vi "cfg upgrade to v2.vi"(11 "Engine Configuration":T11) -> (3 "Engine Configuration out":T1)   [LabVIEW 2013, in "Standard Engine Configuration.lvclass"]
uses:
  Standard Engine Configuration.lvclass
  Supported Timing Sources.ctl
  <vilib>/NI/Tag Bus Module Framework/runtime/error classification.ctl
  Error Actions.ctl
  Engine Configuration.ctl
  Loop Info.ctl
  timing policy.ctl
  Module Specific Configuration.ctl
  Module Decimation.ctl
  Runtime/error responses.ctl
  error options.ctl
  <vilib>/NI/Tag Bus Module Framework/runtime/TBM module execution interface.lvclass
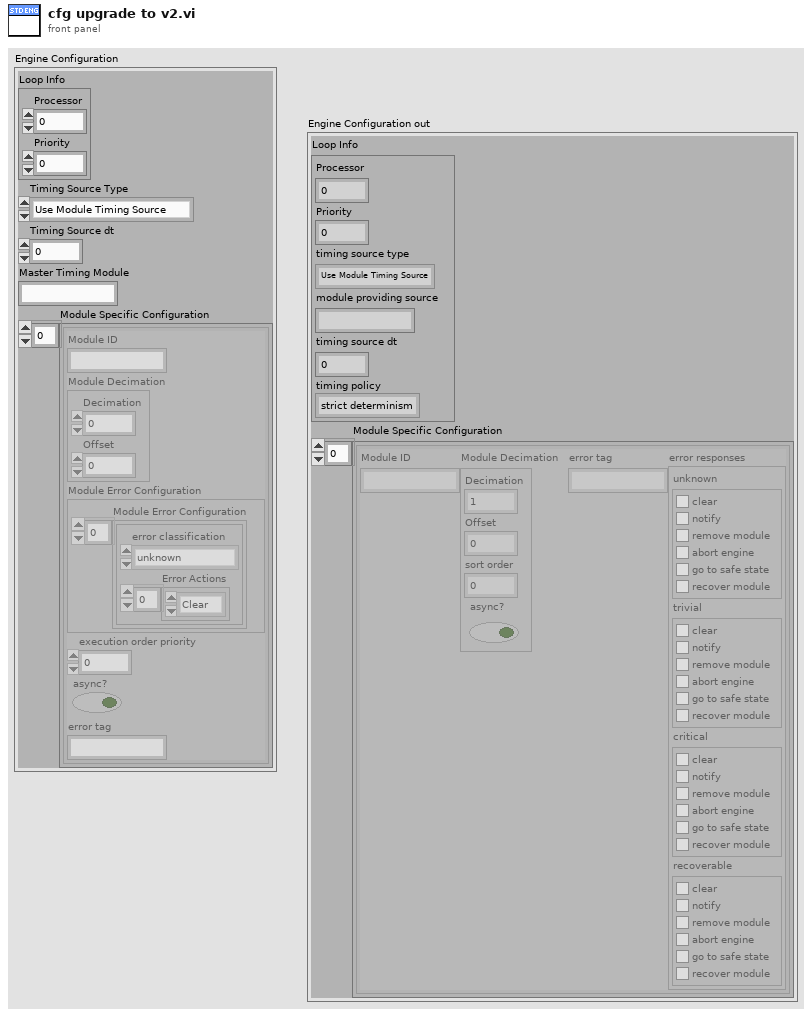
[diagram p1: front panel]
types:
  T1 = typedef "Standard Engine Configuration.lvclass/Engine Configuration.ctl" = cluster{"Loop Info":T2, "Module Specific Configuration":T5[]}
  T2 = typedef "Standard Engine Configuration.lvclass/Loop Info.ctl" = cluster{"Processor":i32, "Priority":i32, "timing source type":T3, "module providing source":string, "timing source dt":u32, "timing policy":T4}
  T3 = typedef "Standard Engine Configuration.lvclass/Supported Timing Sources.ctl" = enum16{"Use Module Timing Source", "1 kHz Clock", "1 MHz Clock", "Synchronize to Scan Engine"}
  T4 = typedef "Standard Engine Configuration.lvclass/timing policy.ctl" = enum16{"strict determinism", "nonblocking", "nondeterministic inline"}
  T5 = typedef "Standard Engine Configuration.lvclass/Module Specific Configuration.ctl" = cluster{"Module ID":string, "Module Decimation":T6, "error tag":string, "error responses":T7}
  T6 = typedef "Standard Engine Configuration.lvclass/Module Decimation.ctl" = cluster{"Decimation":u16, "Offset":u16, "sort order":i32, "async?":bool}
  T7 = typedef "Standard Engine Configuration.lvclass/error responses.ctl" = cluster{"unknown":T8, "trivial":T8, "critical":T8, "recoverable":T8}
  T8 = typedef "Standard Engine Configuration.lvclass/error options.ctl" = cluster{"clear":bool, "notify":bool, "remove module":bool, "abort engine":bool, "go to safe state":bool, "recover module":bool}
  T9 = typedef "TBM module execution interface.lvclass/error classification.ctl" = enum16{"unknown", "none", "trivial", "recoverable", "critical"}
  T10 = typedef "Standard Engine Configuration.lvclass/Error Actions.ctl" = enum16{"Clear", "Notify", "Stop Component", "Stop Engine", "Safe State", "Attempt Recovery"}
  T11 = cluster{"Loop Info":cluster{"Processor":i32, "Priority":i32}, "Timing Source Type":T3, "Timing Source dt":u32, "Master Timing Module":string, "Module Specific Configuration":cluster{"Module ID":string, "Module Decimation":cluster{"Decimation":u16, "Offset":u16}, "Module Error Configuration":cluster{"Module Error Configuration":cluster{"error classification":T9, "Error Actions":T10[]}[]}, "execution order priority":i32, "async?":bool, "error tag":string}[]}
  T12 = cluster{"Module ID":string, "Module Decimation":cluster{"Decimation":u16, "Offset":u16}, "Module Error Configuration":cluster{"Module Error Configuration":cluster{"error classification":T9, "Error Actions":T10[]}[]}, "execution order priority":i32, "async?":bool, "error tag":string}[]
  T13 = cluster{"error classification":T9, "Error Actions":T10[]}[]
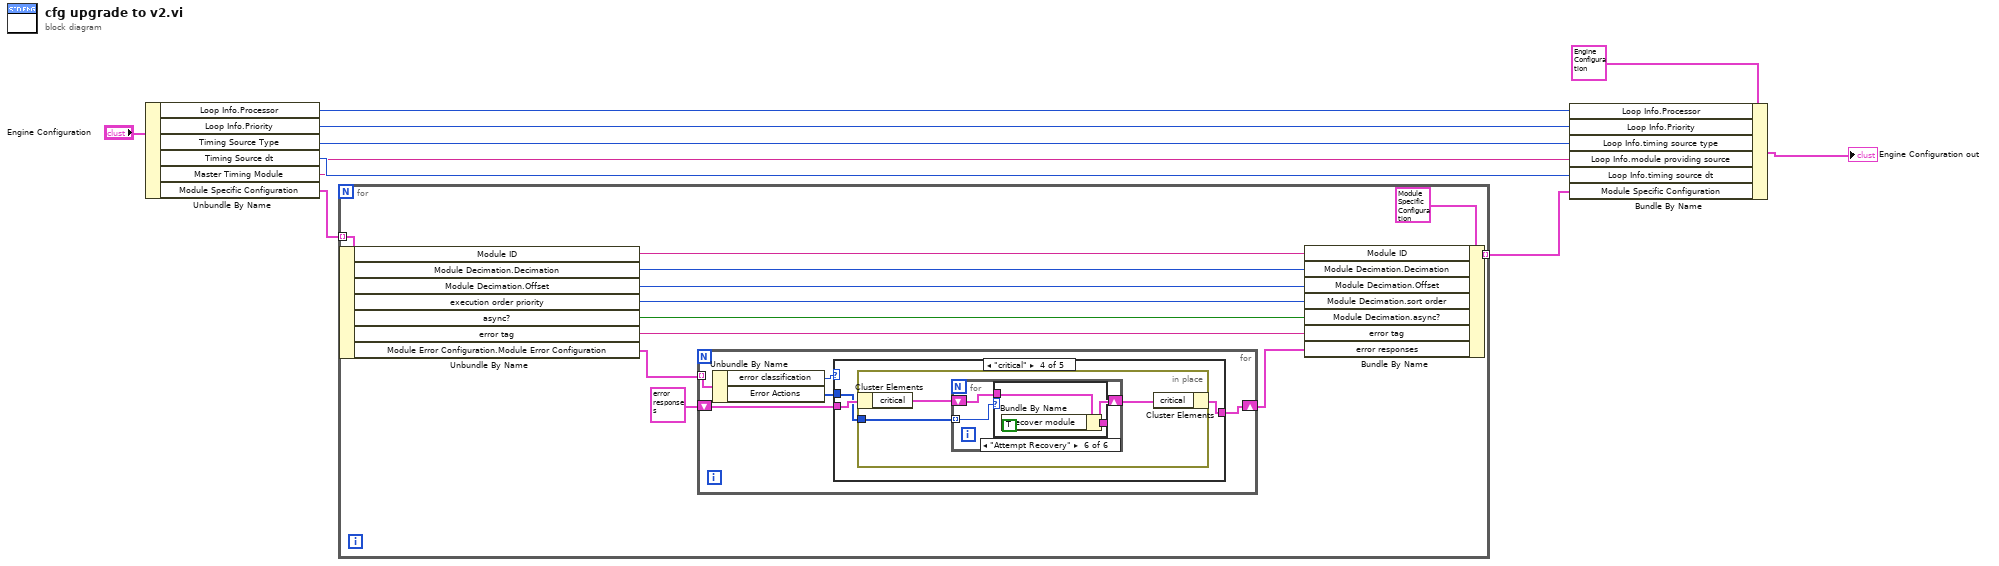
[diagram p0: block diagram]
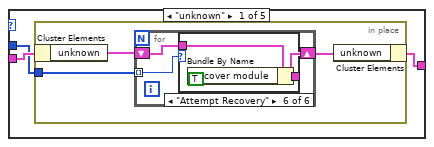
[diagram p2: hidden frame]
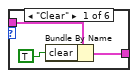
[diagram p3: hidden frame]
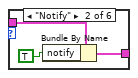
[diagram p4: hidden frame]
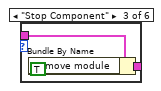
[diagram p5: hidden frame]
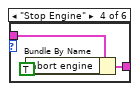
[diagram p6: hidden frame]
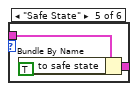
[diagram p7: hidden frame]
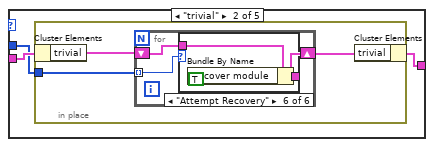
[diagram p8: hidden frame]
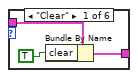
[diagram p9: hidden frame]
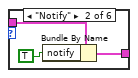
[diagram p10: hidden frame]
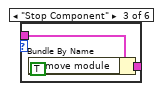
[diagram p11: hidden frame]
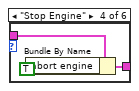
[diagram p12: hidden frame]
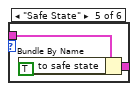
[diagram p13: hidden frame]
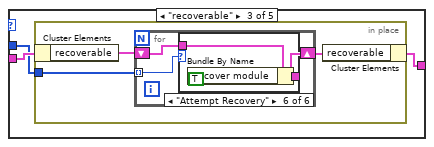
[diagram p14: hidden frame]
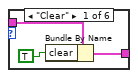
[diagram p15: hidden frame]
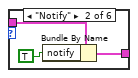
[diagram p16: hidden frame]
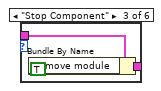
[diagram p17: hidden frame]
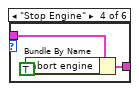
[diagram p18: hidden frame]
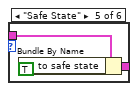
[diagram p19: hidden frame]
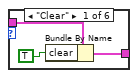
[diagram p20: hidden frame]
diagram:
  n1 = Unbundle By Name("Engine Configuration") -> ("Loop Info.Processor"=w10:i32, "Loop Info.Priority"=w6:i32, "Timing Source Type"=w5:T3, "Timing Source dt"=w4:u32, "Master Timing Module"=w3:string, "Module Specific Configuration"=w1:T12)
  n2 = for {
    tunnel: [w21] -> w2 mode=indexing
    tunnel: w1 -> [w20] mode=indexing
    n3 = Unbundle By Name(w20) -> ("Module ID"=w19:string, "Module Decimation.Decimation"=w14:u16, "Module Decimation.Offset"=w15:u16, "execution order priority"=w16:i32, "async?"=w18:bool, "error tag"=w17:string, "Module Error Configuration.Module Error Configuration"=w13:T13)
    n4 = for {
      tunnel: w13 -> [w27] mode=indexing
      shift-right: [w25] -> w11
      shift-left: T7 {"unknown"={"clear"=FALSE, "notify"=FALSE, "remove module"=FALSE, "abort engine"=FALSE, "go to safe state"=FALSE, "recover module"=FALSE}, "trivial"={"clear"=FALSE, "notify"=FALSE, "remove module"=FALSE, "abort engine"=FALSE, "go to safe state"=FALSE, "recover module"=FALSE}, "critical"={"clear"=FALSE, "notify"=FALSE, "remove module"=FALSE, "abort engine"=FALSE, "go to safe state"=FALSE, "recover module"=FALSE}, "recoverable"={"clear"=FALSE, "notify"=FALSE, "remove module"=FALSE, "abort engine"=FALSE, "go to safe state"=FALSE, "recover module"=FALSE}} ("error responses") -> [w24]
      n5 = Unbundle By Name(w27) -> ("error classification"=w26:T9, "Error Actions"=w23:T10[])
      n6 = case shown="\"critical\"" w26 {
        tunnel: [w29 w56 w83 w110 w136] -> w25
        tunnel: w24 -> [w30 w57 w84 w111 w136]
        tunnel: w23 -> [w28 w55 w82 w109 _]
        frame "unknown" {
          n7 = in-place {
            in-place-border: w28 -> [w31]
            n8 = in-place-cluster #1(w30) -> ("unknown"=w33:T8)
            n9 = for {
              shift-right: [w34] -> w32
              shift-left: w33 -> [w35]
              tunnel: w31 -> [w36] mode=indexing
              n10 = case shown="\"Attempt Recovery\"" w36 {
                tunnel: w35 -> [w39 w42 w45 w48 w51 w54]
                tunnel: [w38 w41 w44 w47 w50 w53] -> w34
                frame "Clear" {
                  n11 = Bundle By Name(cluster=w39, "clear"=TRUE) -> (w38:T8)
                }
                frame "Notify" {
                  n12 = Bundle By Name(cluster=w42, "notify"=TRUE) -> (w41:T8)
                }
                frame "Stop Component" {
                  n13 = Bundle By Name(cluster=w45, "remove module"=TRUE) -> (w44:T8)
                }
                frame "Stop Engine" {
                  n14 = Bundle By Name(cluster=w48, "abort engine"=TRUE) -> (w47:T8)
                }
                frame "Safe State" {
                  n15 = Bundle By Name(cluster=w51, "go to safe state"=TRUE) -> (w50:T8)
                }
                frame "Attempt Recovery" {
                  n16 = Bundle By Name(cluster=w54, "recover module"=TRUE) -> (w53:T8)
                }
              }
            }
            n17 = in-place-cluster #1("unknown"=w32) -> (w29:T7)
          }
        }
        frame "trivial" {
          n18 = in-place {
            in-place-border: w55 -> [w58]
            n19 = in-place-cluster #2(w57) -> ("trivial"=w60:T8)
            n20 = for {
              shift-right: [w61] -> w59
              shift-left: w60 -> [w62]
              tunnel: w58 -> [w63] mode=indexing
              n21 = case shown="\"Attempt Recovery\"" w63 {
                tunnel: w62 -> [w66 w69 w72 w75 w78 w81]
                tunnel: [w65 w68 w71 w74 w77 w80] -> w61
                frame "Clear" {
                  n22 = Bundle By Name(cluster=w66, "clear"=TRUE) -> (w65:T8)
                }
                frame "Notify" {
                  n23 = Bundle By Name(cluster=w69, "notify"=TRUE) -> (w68:T8)
                }
                frame "Stop Component" {
                  n24 = Bundle By Name(cluster=w72, "remove module"=TRUE) -> (w71:T8)
                }
                frame "Stop Engine" {
                  n25 = Bundle By Name(cluster=w75, "abort engine"=TRUE) -> (w74:T8)
                }
                frame "Safe State" {
                  n26 = Bundle By Name(cluster=w78, "go to safe state"=TRUE) -> (w77:T8)
                }
                frame "Attempt Recovery" {
                  n27 = Bundle By Name(cluster=w81, "recover module"=TRUE) -> (w80:T8)
                }
              }
            }
            n28 = in-place-cluster #2("trivial"=w59) -> (w56:T7)
          }
        }
        frame "recoverable" {
          n29 = in-place {
            in-place-border: w82 -> [w85]
            n30 = in-place-cluster #3(w84) -> ("recoverable"=w87:T8)
            n31 = for {
              shift-right: [w88] -> w86
              shift-left: w87 -> [w89]
              tunnel: w85 -> [w90] mode=indexing
              n32 = case shown="\"Attempt Recovery\"" w90 {
                tunnel: w89 -> [w93 w96 w99 w102 w105 w108]
                tunnel: [w92 w95 w98 w101 w104 w107] -> w88
                frame "Clear" {
                  n33 = Bundle By Name(cluster=w93, "clear"=TRUE) -> (w92:T8)
                }
                frame "Notify" {
                  n34 = Bundle By Name(cluster=w96, "notify"=TRUE) -> (w95:T8)
                }
                frame "Stop Component" {
                  n35 = Bundle By Name(cluster=w99, "remove module"=TRUE) -> (w98:T8)
                }
                frame "Stop Engine" {
                  n36 = Bundle By Name(cluster=w102, "abort engine"=TRUE) -> (w101:T8)
                }
                frame "Safe State" {
                  n37 = Bundle By Name(cluster=w105, "go to safe state"=TRUE) -> (w104:T8)
                }
                frame "Attempt Recovery" {
                  n38 = Bundle By Name(cluster=w108, "recover module"=TRUE) -> (w107:T8)
                }
              }
            }
            n39 = in-place-cluster #3("recoverable"=w86) -> (w83:T7)
          }
        }
        frame "critical" {
          n40 = in-place {
            in-place-border: w109 -> [w112]
            n41 = in-place-cluster #4(w111) -> ("critical"=w114:T8)
            n42 = for {
              shift-right: [w115] -> w113
              shift-left: w114 -> [w116]
              tunnel: w112 -> [w117] mode=indexing
              n43 = case shown="\"Attempt Recovery\"" w117 {
                tunnel: w116 -> [w120 w123 w126 w129 w132 w135]
                tunnel: [w119 w122 w125 w128 w131 w134] -> w115
                frame "Clear" {
                  n44 = Bundle By Name(cluster=w120, "clear"=TRUE) -> (w119:T8)
                }
                frame "Notify" {
                  n45 = Bundle By Name(cluster=w123, "notify"=TRUE) -> (w122:T8)
                }
                frame "Stop Component" {
                  n46 = Bundle By Name(cluster=w126, "remove module"=TRUE) -> (w125:T8)
                }
                frame "Stop Engine" {
                  n47 = Bundle By Name(cluster=w129, "abort engine"=TRUE) -> (w128:T8)
                }
                frame "Safe State" {
                  n48 = Bundle By Name(cluster=w132, "go to safe state"=TRUE) -> (w131:T8)
                }
                frame "Attempt Recovery" {
                  n49 = Bundle By Name(cluster=w135, "recover module"=TRUE) -> (w134:T8)
                }
              }
            }
            n50 = in-place-cluster #4("critical"=w113) -> (w110:T7)
          }
        }
        frame "none" {
        }
      }
    }
    n51 = Bundle By Name(cluster=T5 {"Module ID"="", "Module Decimation"={"Decimation"=0, "Offset"=0, "sort order"=0, "async?"=FALSE}, "error tag"="", "error responses"={"unknown"={"clear"=FALSE, "notify"=FALSE, "remove module"=FALSE, "abort engine"=FALSE, "go to safe state"=FALSE, "recover module"=FALSE}, "trivial"={"clear"=FALSE, "notify"=FALSE, "remove module"=FALSE, "abort engine"=FALSE, "go to safe state"=FALSE, "recover module"=FALSE}, "critical"={"clear"=FALSE, "notify"=FALSE, "remove module"=FALSE, "abort engine"=FALSE, "go to safe state"=FALSE, "recover module"=FALSE}, "recoverable"={"clear"=FALSE, "notify"=FALSE, "remove module"=FALSE, "abort engine"=FALSE, "go to safe state"=FALSE, "recover module"=FALSE}}} ("Module Specific Configuration"), "Module ID"=w19, "Module Decimation.Decimation"=w14, "Module Decimation.Offset"=w15, "Module Decimation.sort order"=w16, "Module Decimation.async?"=w18, "error tag"=w17, "error responses"=w11) -> (w21:T5)
  }
  n52 = Bundle By Name(cluster=T1 {"Loop Info"={"Processor"=0, "Priority"=0, "timing source type"=enum."1 MHz Clock", "module providing source"="", "timing source dt"=5000, "timing policy"=enum."nonblocking"}, "Module Specific Configuration"=[]} ("Engine Configuration out"), "Loop Info.Processor"=w10, "Loop Info.Priority"=w6, "Loop Info.timing source type"=w5, "Loop Info.module providing source"=w3, "Loop Info.timing source dt"=w4, "Module Specific Configuration"=w2) -> (→"Engine Configuration out":T1)
